vi "Append Horizontal Line to Report.vi"(0 "report in":refnum<class "NI_report.lvclass">, 1 "size (default)":i32=1, 2 "MS Office parameters":T2, 5 "align (default)":T1, 9 "width (100=default)":dbl=100.0 format="%.2f", 11 "error in (no error)":errorcluster, 12 "width units":enum16{"Pixels", "Percentage"}(ring)=enum."Percentage", 13 "noshade (F)":bool) -> (4 "report out":refnum<class "NI_report.lvclass">, 15 "error out":errorcluster)   [LabVIEW 2020, in "NI_report.lvclass"]
doc: "Creates a horizontal rule in an HTML report."
uses:
  <vilib>/Utility/NIReport.llb/NI_report.lvclass
  <vilib>/Utility/NIReport.llb/HTML Report Text Alignment.ctl
  <vilib>/Utility/NIReport.llb/NI_ReportGenerationCore.lvlib
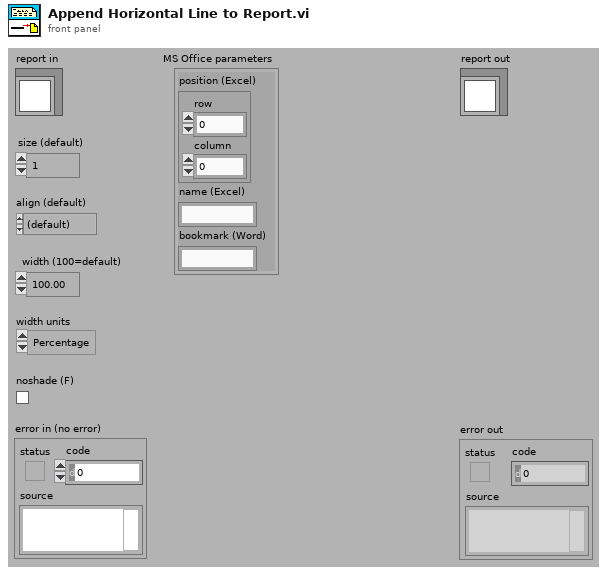
[diagram p1: front panel]
types:
  T1 = typedef "NI_ReportGenerationCore.lvlib/HTML Report Text Alignment.ctl" = enum16{"(default)", "LEFT", "CENTER", "RIGHT"}
  T2 = cluster{"position (Excel)":cluster{"row":i32, "column":i32}, "name (Excel)":string, "bookmark (Word)":string}
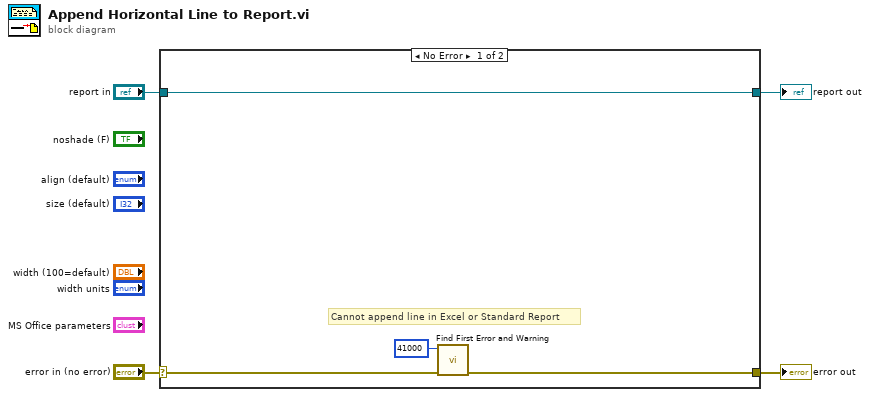
[diagram p0: block diagram]
diagram:
  n1 = case shown="No Error" "error in (no error)" {
    selector: "error in (no error)" -> [w6 w10]
    tunnel: [w5 w10] -> w3
    tunnel: [w8 w9] -> w1
    tunnel: "report in" -> [w8 w9]
    frame No Error {
      # "Cannot append line in Excel or Standard Report"
      n2 = call <vilib>:"Find First Error and Warning.vi"("error in (no error)"=w6, "error code"=41000) -> ("error out"=w5:errorcluster)  [unwired: 1 in, 4 out]
    }
    frame Error {
    }
  }
  "error out" <- w3
  "report out" <- w1
